vi "nanoVoltRead_LightCurrentControl.vi"() -> ()   [LabVIEW 2014]
uses:
  <vilib>/Utility/file.llb/Write To Spreadsheet File (string).vi
  subvi/Keithley 24XX/Keithley 24XX.lvlib
panel:
  out "error out":errorcluster
  out "Current Out (A)":sgl[](array[numeric])
  out "Voltage Out (V)":sgl[](array[numeric])
  out "Ready":bool
  out "Current Setpoint (A)":dbl
  in  "VISA resource name":refnum<visa-resource-name>="GPIB0::24::INSTR"
  in  "Time2\n(s)":dbl[](array[numeric])
  in  "Current\n(mA)":dbl[](array[numeric])
  in  "Filename Label (optional)":string
  in  "Channel\n(0,1,2)":dbl[](array[numeric])
  out "Light Intensity":dbl
  in  "Time1\n(s)":dbl[](array[numeric])
  in  "Intensity\n(0-100%)":dbl[](array[numeric])
  in  "Baud Rate":dbl=57600.0
  in  "Light Port":refnum<visa-resource-name>="COM4"
  in  "Previous Top T":dbl
  in  "Temp Rate (s)":dbl=0.25
  in  "Previous Delta T":dbl
  in  "T read time":dbl
  out "Temp2 (C)":dbl format="%#.4g"
  out "Temp1 (C)":dbl format="%#.4g"
  out "Delta T (C)":dbl format="%#.4g"
  in  "Temp2 Port":tag="Dev2"
  in  "Temp1 Port":tag="Dev1"
  in  "Rate (0.1 - 5)":string="5"
  out "Time (s)":dbl caption="Elapsed Time (s)"
  out "XY Graph":cluster{dbl[], dbl[]}[](graph)
  in  "file (use dialog)":path=path "C:/Users/probe_station/Desktop/nanoVolt"
  out "Measurement Number":i32
  in  "stop":bool
  out "Voltage(uV)":dbl
  in  "GPIB\nAddress":string="9"
  # "Keithly 2401 Controls"
  # "Keithley Model 2182A Nanovoltmeter Read\n2014-03-19\nMichael Kabatek & David Ellsworth\nCSU Magnetics Lab"
  # "Ignore These"
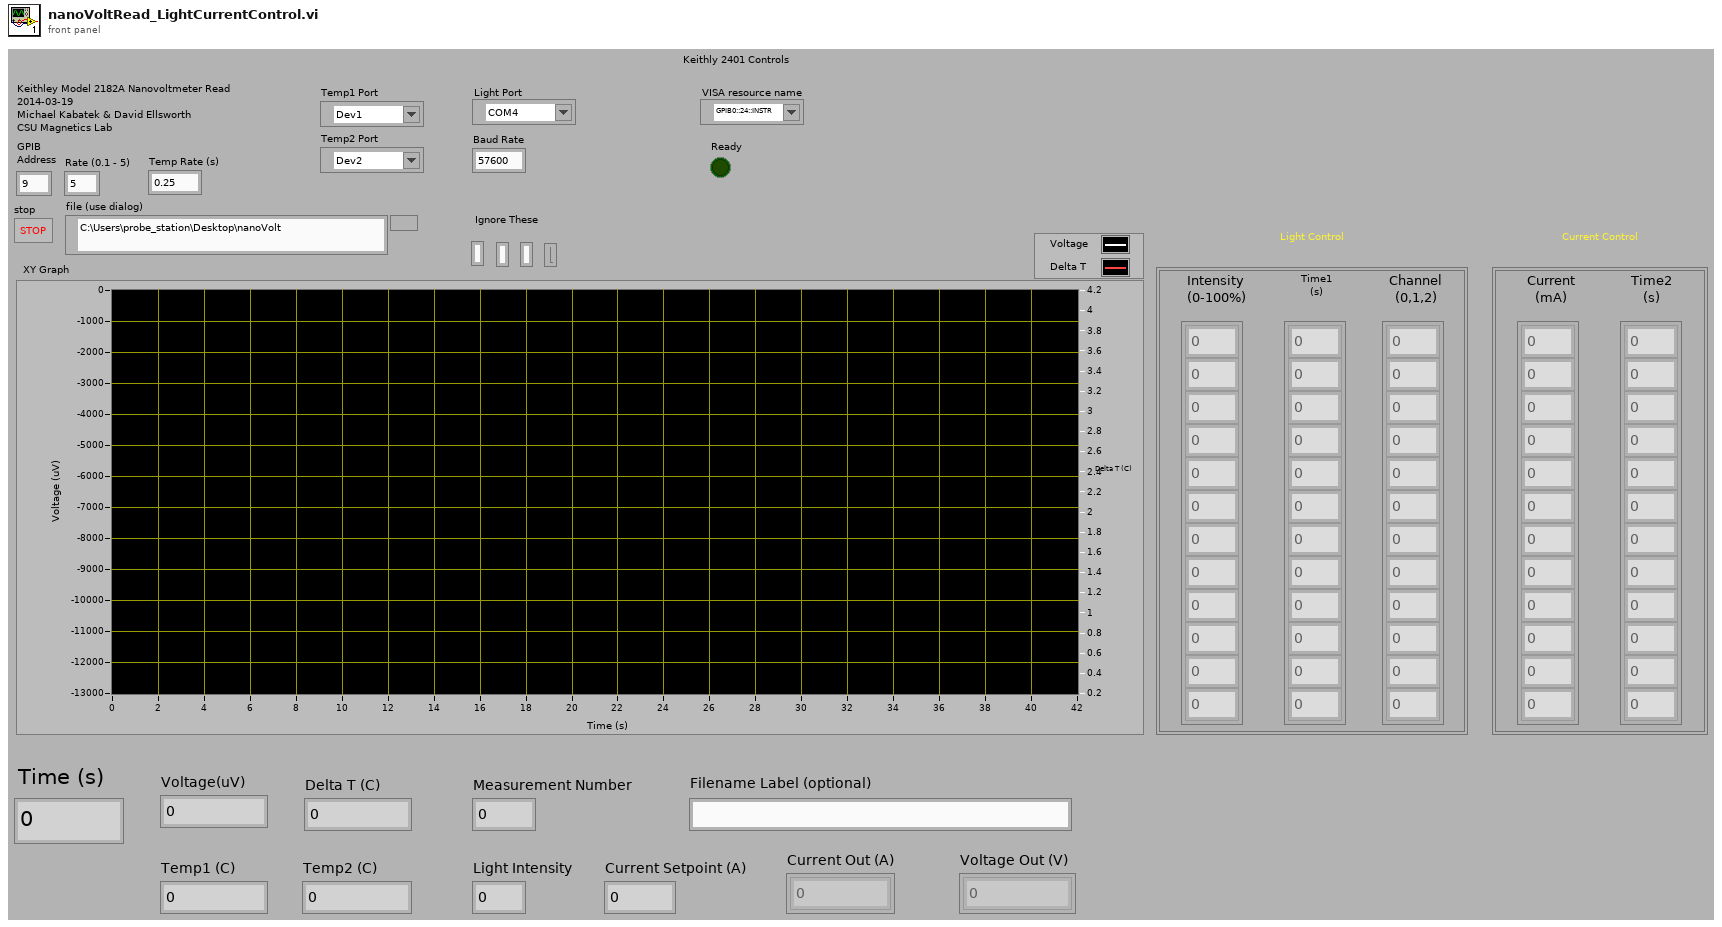
[diagram p1: front panel]
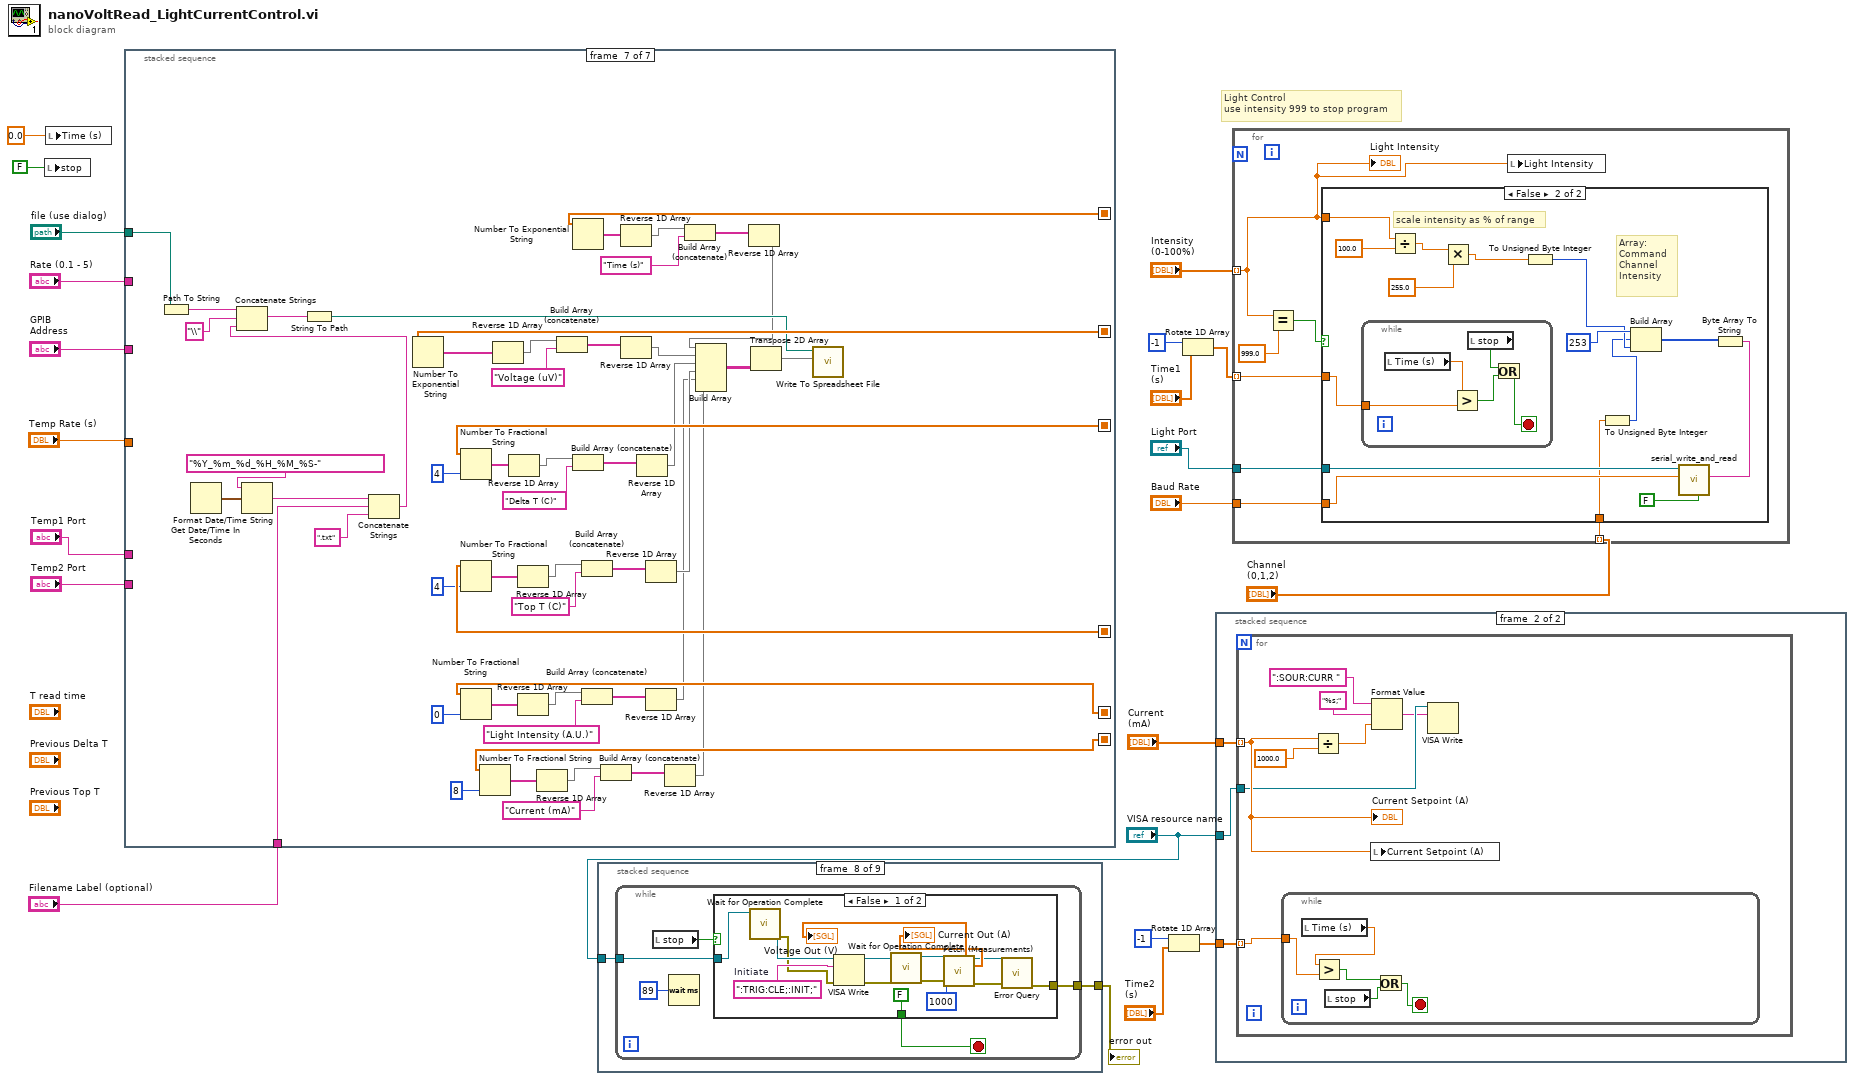
[diagram p0: block diagram]
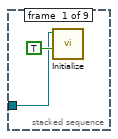
[diagram p2: hidden frame]
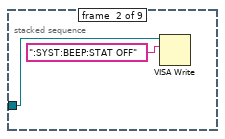
[diagram p3: hidden frame]
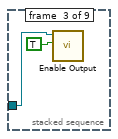
[diagram p4: hidden frame]
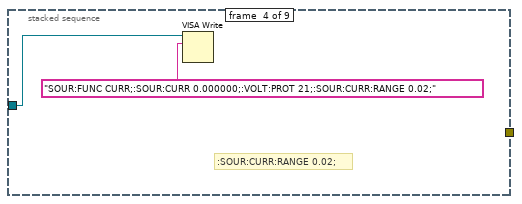
[diagram p5: hidden frame]
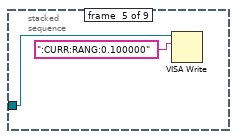
[diagram p6: hidden frame]
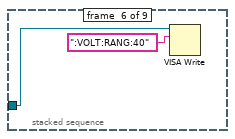
[diagram p7: hidden frame]
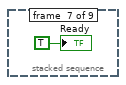
[diagram p8: hidden frame]
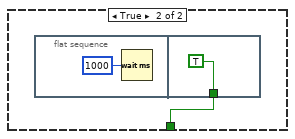
[diagram p9: hidden frame]
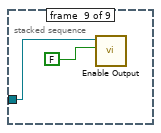
[diagram p10: hidden frame]
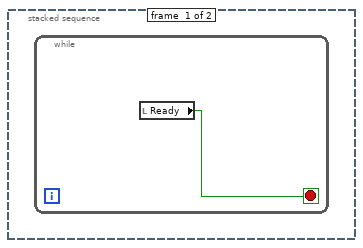
[diagram p11: hidden frame]
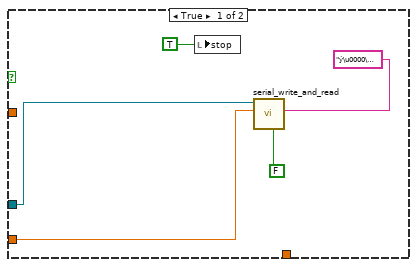
[diagram p12: hidden frame]
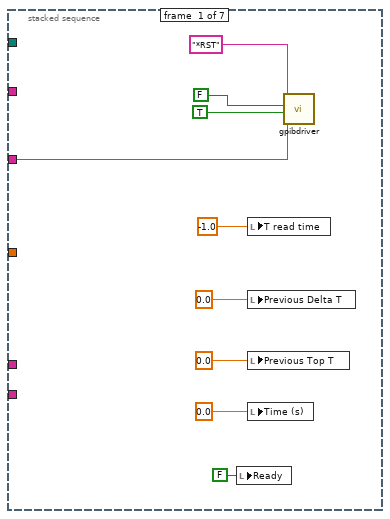
[diagram p13: hidden frame]
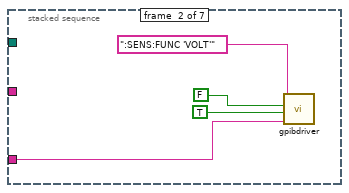
[diagram p14: hidden frame]
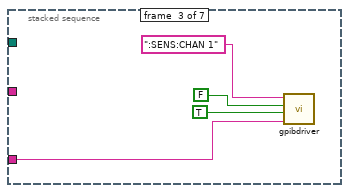
[diagram p15: hidden frame]
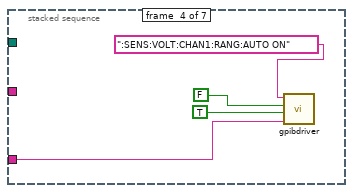
[diagram p16: hidden frame]
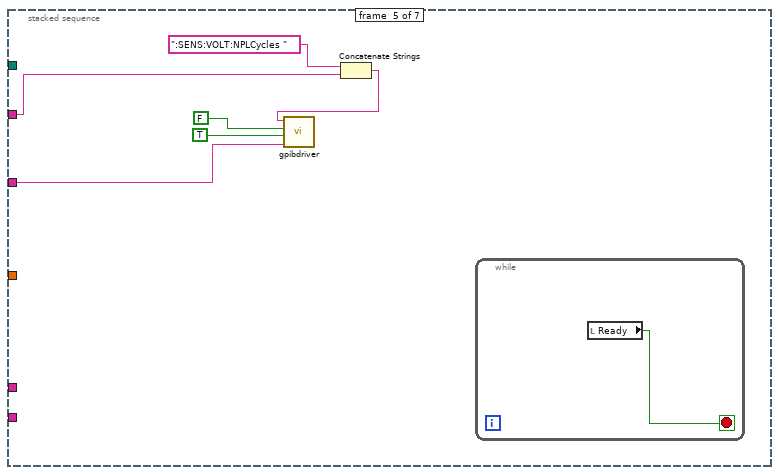
[diagram p17: hidden frame]
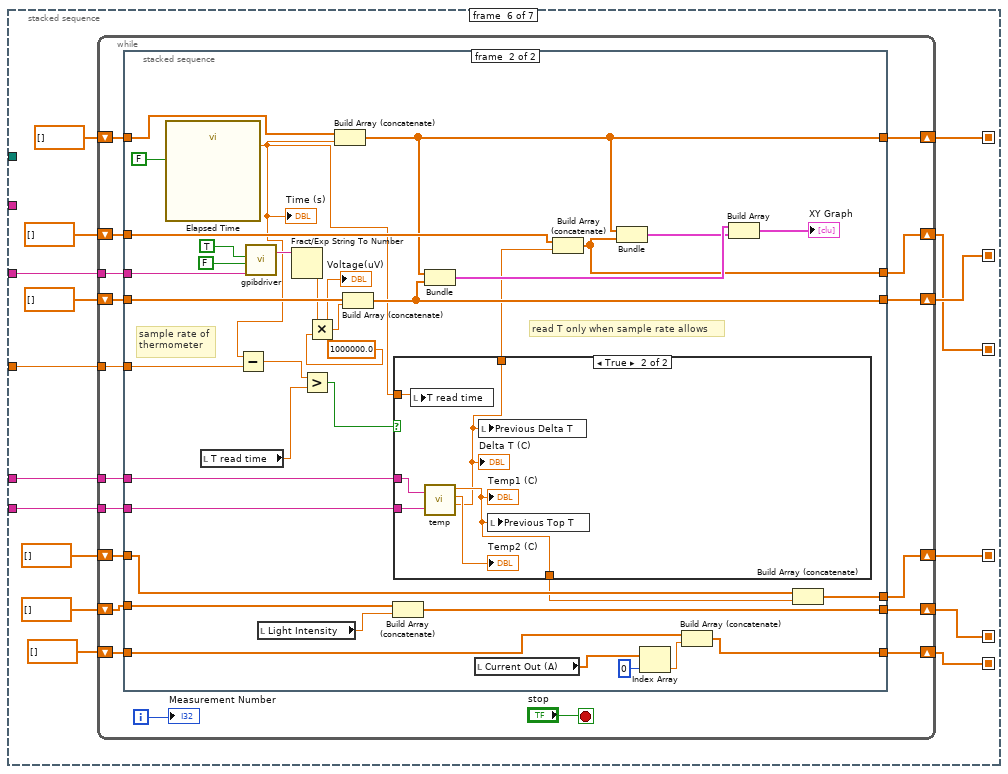
[diagram p18: hidden frame]
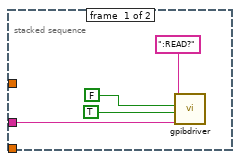
[diagram p19: hidden frame]
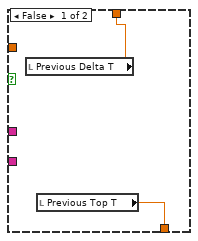
[diagram p20: hidden frame]
diagram:
  # "Light Control\nuse intensity 999 to stop program"
  n1 = local write "stop"(FALSE ("stop")) -> ()
  n2 = local write "Time (s)"(0.0 ("Time (s)")) -> ()
  n3 = stacked-sequence {
    seq-local: [_ _ _ _ _ w64 _] -> [_ _ _ _ _ _ w177]
    seq-local: [_ _ _ _ _ w62 _] -> [_ _ _ _ _ _ w170]
    seq-local: [_ _ _ _ _ w59 _] -> [_ _ _ _ _ _ w174]
    seq-local: [_ _ _ _ _ w56 _] -> [_ _ _ _ _ _ w172]
    seq-local: [_ _ _ _ _ w53 _] -> [_ _ _ _ _ _ w143]
    seq-local: [_ _ _ _ _ w51 _] -> [_ _ _ _ _ _ w134]
    tunnel: "GPIB\nAddress" -> [w28 w32 w36 w40 w47 w66 _]
    tunnel: "file (use dialog)" -> [_ _ _ _ _ _ w179]
    tunnel: "Temp1 Port" -> [_ _ _ _ _ w61 _]
    tunnel: "Temp2 Port" -> [_ _ _ _ _ w60 _]
    tunnel: "Rate (0.1 - 5)" -> [_ _ _ _ w44 _ _]
    tunnel: "Temp Rate (s)" -> [_ _ _ _ _ w57 _]
    tunnel: "Filename Label (optional)" -> [_ _ _ _ _ _ w140]
    frame #0 {
      n4 = local write "Ready"(FALSE ("Ready")) -> ()
      n5 = local write "T read time"(-1.0 ("read T")) -> ()
      n6 = local write "Previous Delta T"(0.0 ("Previous T")) -> ()
      n7 = local write "Previous Top T"(0.0 ("Previous Top T")) -> ()
      n8 = local write "Time (s)"(0.0 ("Time (s)")) -> ()
      n9 = call "gpibdriver.vi"("Characters to Write"="*RST", "Read"=FALSE, "Write"=TRUE ("Write 3"), "GPIB\nAddress"=w28) -> ()  [unwired: 2 in, 1 out]
    }
    frame #1 {
      n10 = call "gpibdriver.vi"("Characters to Write"=":SENS:FUNC 'VOLT'", "Read"=FALSE, "Write"=TRUE ("Write 3"), "GPIB\nAddress"=w32) -> ()  [unwired: 2 in, 1 out]
    }
    frame #2 {
      n11 = call "gpibdriver.vi"("Characters to Write"=":SENS:CHAN 1", "Read"=FALSE, "Write"=TRUE ("Write 3"), "GPIB\nAddress"=w36) -> ()  [unwired: 2 in, 1 out]
    }
    frame #3 {
      n12 = call "gpibdriver.vi"("Characters to Write"=":SENS:VOLT:CHAN1:RANG:AUTO ON", "Read"=FALSE, "Write"=TRUE ("Write 3"), "GPIB\nAddress"=w40) -> ()  [unwired: 2 in, 1 out]
    }
    frame #4 {
      n13 = Concatenate Strings(":SENS:VOLT:NPLCycles " ("Characters to Write"), w44) -> (w45:string)
      n14 = call "gpibdriver.vi"("Characters to Write"=w45, "Read"=FALSE, "Write"=TRUE ("Write 3"), "GPIB\nAddress"=w47) -> ()  [unwired: 2 in, 1 out]
      n15 = while {
        stop <- w50 stop-if-true
        n16 = local read "Ready"() -> (w50:bool)
      }
    }
    frame #5 {
      n17 = while {
        tunnel: w66 -> [w84]
        shift-right: [w82] -> w64
        shift-left: dbl[] [] -> [w81]
        shift-right: [w78] -> w62
        shift-left: dbl[] [] -> [w79]
        tunnel: w61 -> [w77]
        tunnel: w60 -> [w76]
        shift-right: [w75] -> w59
        shift-left: dbl[] [] -> [w74]
        tunnel: w57 -> [w73]
        shift-right: [w71] -> w56
        shift-left: dbl[] [] -> [w72]
        shift-right: [w69] -> w53
        shift-left: dbl[] [] -> [w70]
        shift-right: [w67] -> w51
        shift-left: dbl[] [] -> [w68]
        i -> [w80]
        stop <- "stop" stop-if-true
        n18 = stacked-sequence {
          tunnel: w84 -> [w85 w122]
          tunnel: [_ w117] -> w82
          tunnel: w81 -> [_ w121]
          tunnel: w79 -> [_ w119]
          tunnel: [_ w109] -> w78
          tunnel: w77 -> [_ w116]
          tunnel: w76 -> [_ w115]
          tunnel: [_ w111] -> w75
          tunnel: w74 -> [_ w112]
          tunnel: w73 -> [_ w103]
          tunnel: w72 -> [_ w102]
          tunnel: [_ w100] -> w71
          tunnel: w70 -> [_ w99]
          tunnel: [_ w97] -> w69
          tunnel: w68 -> [_ w93]
          tunnel: [_ w92] -> w67
          frame #0 {
            n19 = call "gpibdriver.vi"("Characters to Write"=":READ?", "Read"=FALSE, "Write"=TRUE ("Write 3"), "GPIB\nAddress"=w85) -> ()  [unwired: 2 in, 1 out]
          }
          frame #1 {
            # "read T only when sample rate allows"
            # "sample rate of\nthermometer"
            n20 = call "Elapsed Time"("Auto Reset"=FALSE) -> ("Elapsed Time (s)"=w106:dbl)  [unwired: 11 in, 7 out]
            "Time (s)" <- w106
            n21 = local read "T read time"() -> (w104:dbl)
            n22 = Subtract(x=w106, y=w103) -> (x-y=w105:dbl)
            n23 = call "gpibdriver.vi"("Read"=TRUE, "Write"=FALSE ("Write 3"), "GPIB\nAddress"=w122) -> ("Characters Read"=w120:string)  [unwired: 3 in]
            n24 = local read "Light Intensity"() -> (w98:dbl)
            n25 = Fract/Exp String To Number(string=w120) -> (number=w96:dbl)  [unwired: 3 in, 1 out]
            n26 = Greater?(x=w105, y=w104) -> (0:w107:bool)
            n27 = Multiply(x=w96, y=1000000.0) -> (x*y=w94:dbl)
            "Voltage(uV)" <- w94
            n28 = Build Array (concatenate)(w119, w106) -> (w109:dbl[])
            n29 = Build Array (concatenate)(w121, w94) -> (w117:dbl[])
            n30 = Build Array (concatenate)(w99, w98) -> (w97:dbl[])
            n31 = case shown="True" w107 {
              tunnel: w116 -> [_ w131]
              tunnel: w115 -> [_ w130]
              tunnel: [w126 w127] -> w113
              tunnel: w106 -> [_ w132]
              tunnel: [w125 w129] -> w101
              frame False {
                n32 = local read "Previous Delta T"() -> (w126:dbl)
                n33 = local read "Previous Top T"() -> (w125:dbl)
              }
              frame True {
                n34 = local write "T read time"(w132) -> ()
                n35 = call "temp.vi"("Temp2 (Bottom) Port"=w130, "Temp1 (Top) Port"=w131) -> ("Delta T"=w127:dbl, "Bottom"=→"Temp2 (C)":dbl, "Top"=w129:dbl)  [unwired: 2 out]
                "Delta T (C)" <- w127
                "Temp1 (C)" <- w129
                n36 = local write "Previous Delta T"(w127) -> ()
                n37 = local write "Previous Top T"(w129) -> ()
              }
            }
            n38 = Bundle(w109, w117) -> (w114:cluster{dbl[], dbl[]})  [unwired: 1 in]
            n39 = local read "Current Out (A)"() -> (w91:sgl[])
            n40 = Build Array (concatenate)(w112, w113) -> (w111:dbl[])
            n41 = Bundle(w109, w111) -> (w108:cluster{dbl[], dbl[]})  [unwired: 1 in]
            n42 = Index Array(array=w91, index=0) -> (element=w89:sgl)
            n43 = Build Array (concatenate)(w93, w89) -> (w92:dbl[])
            n44 = Build Array(w114, w108) -> (→"XY Graph":cluster{dbl[], dbl[]}[])
            n45 = Build Array (concatenate)(w102, w101) -> (w100:dbl[])
          }
        }
        "Measurement Number" <- w80
      }
    }
    frame #6 {
      n46 = Path To String(path=w179) -> (string=w182:string)
      n47 = Get Date/Time In Seconds() -> (seconds since 1Jan1904=w185:timestamp)
      n48 = Format Date/Time String(time format string (%c)="%Y_%m_%d_%H_%M_%S-", seconds (now)=w185) -> (date/time string=w183:string)  [unwired: 1 in]
      n49 = Concatenate Strings(w183, w140, ".txt" ("string")) -> (w178:string)
      n50 = Concatenate Strings(w182, "\\" ("string"), w178) -> (w180:string)
      n51 = String To Path(string=w180) -> (path=w176:path)
      n52 = Number To Exponential String(number=w177) -> (E-format string=w164:string[])  [unwired: 3 in]
      n53 = Number To Fractional String(number=w174, precision (6)=i16 4) -> (F-format string=w159:string[])  [unwired: 2 in]
      n54 = Number To Fractional String(number=w172, precision (6)=i16 4) -> (F-format string=w152:string[])  [unwired: 2 in]
      n55 = Number To Fractional String(number=w143, precision (6)=i16 0) -> (F-format string=w144:string[])  [unwired: 2 in]
      n56 = Number To Fractional String(number=w134, precision (6)=i16 8) -> (F-format string=w135:string[])  [unwired: 2 in]
      n57 = Reverse 1D Array(array=w164) -> (reversed array=w163:string[])
      n58 = Reverse 1D Array(array=w159) -> (reversed array=w158:string[])
      n59 = Reverse 1D Array(array=w152) -> (reversed array=w154:string[])
      n60 = Reverse 1D Array(array=w144) -> (reversed array=w146:string[])
      n61 = Reverse 1D Array(array=w135) -> (reversed array=w137:string[])
      n62 = Build Array (concatenate)(w163, "Voltage (uV)") -> (w162:string[])
      n63 = Number To Exponential String(number=w170) -> (E-format string=w168:string[])  [unwired: 3 in]
      n64 = Build Array (concatenate)(w158, "Delta T (C)") -> (w160:string[])
      n65 = Build Array (concatenate)(w154, "Top T (C)") -> (w155:string[])
      n66 = Build Array (concatenate)(w146, "Light Intensity (A.U.)") -> (w147:string[])
      n67 = Build Array (concatenate)(w137, "Current (mA)") -> (w138:string[])
      n68 = Reverse 1D Array(array=w168) -> (reversed array=w167:string[])
      n69 = Reverse 1D Array(array=w162) -> (reversed array=w161:string[])
      n70 = Reverse 1D Array(array=w160) -> (reversed array=w157:string[])
      n71 = Reverse 1D Array(array=w155) -> (reversed array=w151:string[])
      n72 = Reverse 1D Array(array=w147) -> (reversed array=w142:string[])
      n73 = Reverse 1D Array(array=w138) -> (reversed array=w133:string[])
      n74 = Build Array (concatenate)(w167, "Time (s)") -> (w166:string[])
      n75 = Reverse 1D Array(array=w166) -> (reversed array=w165:string[])
      n76 = Build Array(w165, w161, w157, w151, w142, w133) -> (w169:string[][])
      n77 = Transpose 2D Array(2D array=w169) -> (transposed array=w175:string[][])
      n78 = call-poly <vilib>:"Write To Spreadsheet File.vi"("2D data"=w175, "file path (dialog if empty)"=w176) -> ()  [unwired: 6 in, 1 out]
    }
  }
  n79 = stacked-sequence {
    tunnel: "VISA resource name" -> [w186 w188 w190 w193 w194 w196 _ w200 w224]
    tunnel: [_ _ _ _ _ _ _ w199 _] -> w1
    frame #0 {
      n80 = call "Initialize.vi"("Reset (True)"=TRUE, "VISA resource name"=w186) -> ()  [unwired: 8 in, 2 out]
    }
    frame #1 {
      n81 = VISA Write(VISA resource name=w188, write buffer=":SYST:BEEP:STAT OFF") -> ()  [unwired: 1 in, 3 out]
    }
    frame #2 {
      n82 = call "Enable Output.vi"("Enable Output (T: Enable)"=TRUE, "VISA resource name"=w190) -> ()  [unwired: 8 in, 2 out]
    }
    frame #3 {
      # ":SOUR:CURR:RANGE 0.02;"
      n83 = VISA Write(VISA resource name=w193, write buffer="SOUR:FUNC CURR;:SOUR:CURR 0.000000;:VOLT:PROT 21;:SOUR:CURR:RANGE 0.02;") -> ()  [unwired: 1 in, 3 out]
    }
    frame #4 {
      n84 = VISA Write(VISA resource name=w194, write buffer=":CURR:RANG:0.100000") -> ()  [unwired: 1 in, 3 out]
    }
    frame #5 {
      n85 = VISA Write(VISA resource name=w196, write buffer=":VOLT:RANG:40") -> ()  [unwired: 1 in, 3 out]
    }
    frame #6 {
      "Ready" <- TRUE ("Ready")
    }
    frame #7 {
      n86 = while {
        tunnel: w200 -> [w205]
        tunnel: [w201] -> w199
        stop <- w202 stop-if-true
        n87 = local read "stop"() -> (w204:bool)
        n88 = Wait (ms)(milliseconds to wait=u32 89) -> ()  [unwired: 1 out]
        n89 = case shown="False" w204 {
          tunnel: w205 -> [w217 _]
          tunnel: [FALSE w221] -> w202
          tunnel: [w206 _] -> w201
          frame False {
            w220 = ":TRIG:CLE;:INIT;"  # Initiate
            n90 = call "Wait for Operation Complete.vi"("VISA resource name"=w217) -> ("error out"=w210:errorcluster, "VISA resource name out"=w216:refnum<visa-resource-name>)  [unwired: 9 in]
            n91 = VISA Write(VISA resource name=w216, write buffer=w220, error in (no error)=w210) -> (VISA resource name out=w215:refnum<visa-resource-name>, error out=w212:errorcluster)  [unwired: 1 out]
            n92 = call "Wait for Operation Complete.vi"("error in (no error)"=w212, "VISA resource name"=w215) -> ("error out"=w211:errorcluster, "VISA resource name out"=w214:refnum<visa-resource-name>)  [unwired: 8 in]
            n93 = call "Fetch (Measurements).vi"("VISA resource name"=w214, "Timeout (10000 ms)"=1000, "error in (no error)"=w211) -> ("Voltage"=→"Voltage Out (V)":sgl[], "VISA resource name out"=w208:refnum<visa-resource-name>, "Current"=→"Current Out (A)":sgl[], "error out"=w209:errorcluster)  [unwired: 6 in, 3 out]
            n94 = call "Error Query.vi"("error in (no error)"=w209, "VISA resource name"=w208) -> ("error out"=w206:errorcluster)  [unwired: 6 in, 3 out]
          }
          frame True {
            n95 = flat-sequence {
              tunnel: [TRUE] -> w221
              frame #0 {
                n96 = Wait (ms)(milliseconds to wait=u32 1000) -> ()  [unwired: 1 out]
              }
              frame #1 {
              }
            }
          }
        }
      }
    }
    frame #8 {
      n97 = call "Enable Output.vi"("Enable Output (T: Enable)"=FALSE, "VISA resource name"=w224) -> ()  [unwired: 8 in, 2 out]
    }
  }
  "error out" <- w1
  n98 = Rotate 1D Array(1:"Time2\n(s)", 2:-1 ("n")) -> (0:w3:dbl[])
  n99 = Rotate 1D Array(1:"Time1\n(s)", 2:-1 ("n")) -> (0:w9:dbl[])
  n100 = stacked-sequence {
    tunnel: "Current\n(mA)" -> [_ w229]
    tunnel: w3 -> [_ w228]
    tunnel: "VISA resource name" -> [_ w227]
    frame #0 {
      n101 = while {
        stop <- w226 stop-if-true
        n102 = local read "Ready"() -> (w226:bool)
      }
    }
    frame #1 {
      n103 = for {
        tunnel: w229 -> [w235] mode=indexing
        tunnel: w228 -> [w237] mode=indexing
        tunnel: w227 -> [w234]
        n104 = while {
          tunnel: w237 -> [w241]
          stop <- w242 stop-if-true
          n105 = local read "Time (s)"() -> (w240:dbl)
          n106 = Greater?(x=w240, y=w241) -> (0:w238:bool)
          n107 = local read "stop"() -> (w239:bool)
          n108 = Or(x=w238, y=w239) -> (x .or. y?=w242:bool)
        }
        n109 = Divide(x=w235, y=1000.0) -> (x/y=w232:dbl)
        n110 = local write "Current Setpoint (A)"(w235) -> ()
        n111 = Format Value(string ("")=":SOUR:CURR " ("string"), format string="%s;", value (0)=w232) -> (output string=w230:string)
        n112 = VISA Write(VISA resource name=w234, write buffer=w230) -> ()  [unwired: 1 in, 3 out]
        "Current Setpoint (A)" <- w235
      }
    }
  }
  n113 = for {
    tunnel: "Intensity\n(0-100%)" -> [w243] mode=indexing
    tunnel: w9 -> [w247] mode=indexing
    tunnel: "Light Port" -> [w249]
    tunnel: "Baud Rate" -> [w248]
    tunnel: "Channel\n(0,1,2)" -> [w244] mode=indexing
    n114 = Equal?(x=w243, y=999.0) -> (x = y?=w246:bool)
    n115 = case shown="False" w246 {
      tunnel: w249 -> [w253 w261]
      tunnel: w248 -> [w252 w260]
      tunnel: w247 -> [_ w259]
      tunnel: w243 -> [_ w258]
      tunnel: w244 -> [_ w256]
      frame True {
        n116 = local write "stop"(TRUE ("stop")) -> ()
        n117 = call "serial_write_and_read.vi"("VISA resource name"=w253, "baud rate"=w252, "read"=FALSE, "string to write"="ý\u0000\u0000") -> ()  [unwired: 6 in, 1 out]
      }
      frame False {
        # "Array:\nCommand\nChannel\nIntensity"
        # "scale intensity as % of range"
        n118 = while {
          tunnel: w259 -> [w271]
          stop <- w274 stop-if-true
          n119 = local read "Time (s)"() -> (w272:dbl)
          n120 = Greater?(x=w272, y=w271) -> (0:w270:bool)
          n121 = local read "stop"() -> (w273:bool)
          n122 = Or(x=w273, y=w270) -> (x .or. y?=w274:bool)
        }
        n123 = Divide(x=w258, y=100.0) -> (x/y=w268:dbl)
        n124 = Multiply(x=w268, y=255.0) -> (x*y=w266:dbl)
        n125 = To Unsigned Byte Integer(number=w266) -> (unsigned 8bit integer=w257:u8)
        n126 = To Unsigned Byte Integer(number=w256) -> (unsigned 8bit integer=w255:u8)
        n127 = Build Array(u8 253 ("element"), w255, w257) -> (w264:u8[])
        n128 = Byte Array To String(unsigned byte array=w264) -> (string=w263:string)
        n129 = call "serial_write_and_read.vi"("VISA resource name"=w261, "baud rate"=w260, "read"=FALSE, "string to write"=w263) -> ()  [unwired: 6 in, 1 out]
      }
    }
    n130 = local write "Light Intensity"(w243) -> ()
    "Light Intensity" <- w243
  }
